vi "Auto Rally Point Calculations.vi"(8 "Rally Point Offset":dbl=24.0, 9 "Depth":dbl=115.0, 10 "Goal Target":T1, 11 "Starting Position":T2) -> (2 "Distance":dbl=294.3908965983833, 3 "Angle":dbl=67.00585386224785)   [LabVIEW 2015]
uses:
  Defense Position.ctl
  Goal Selection.ctl
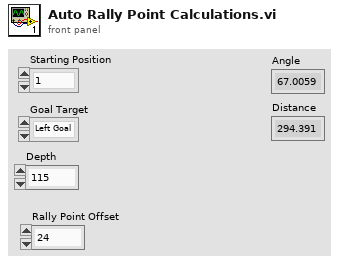
[diagram p1: front panel]
types:
  T1 = typedef "Goal Selection.ctl" = enum16{"Left Goal", "Right Goal"}
  T2 = typedef "Defense Position.ctl" = enum16{"1", "2", "3", "4", "5"}
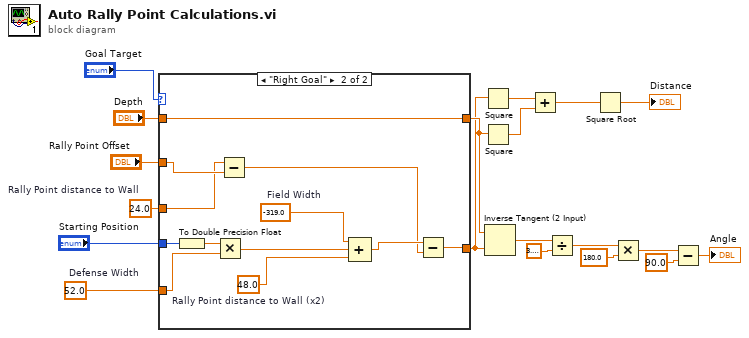
[diagram p0: block diagram]
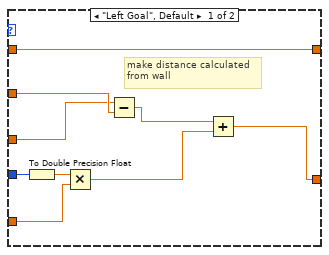
[diagram p2: hidden frame]
diagram:
  w1 = 24.0  # Rally Point distance to Wall
  w12 = 52.0  # Defense Width
  n1 = case shown="\"Right Goal\"" "Goal Target" {
    tunnel: "Depth" -> [w27 w39]
    tunnel: [w23 w31] -> w13
    tunnel: [w27 w39] -> w14
    tunnel: w12 -> [w26 w38]
    tunnel: "Starting Position" -> [w25 w36]
    tunnel: "Rally Point Offset" -> [w21 w33]
    tunnel: w1 -> [w20 w32]
    frame "Left Goal", Default {
      # "make distance calculated\nfrom wall"
      n2 = To Double Precision Float(number=w25) -> (double precision float=w28:dbl)
      n3 = Multiply(x=w28, y=w26) -> (x*y=w24:dbl)
      n4 = Subtract(x=w20, y=w21) -> (x-y=w22:dbl)
      n5 = Add(x=w22, y=w24) -> (x+y=w23:dbl)
    }
    frame "Right Goal" {
      w35 = 48.0  # Rally Point distance to Wall (x2)
      w37 = -319.0  # Field Width
      n6 = To Double Precision Float(number=w36) -> (double precision float=w40:dbl)
      n7 = Multiply(x=w40, y=w38) -> (x*y=w34:dbl)
      n8 = Subtract(x=w32, y=w33) -> (x-y=w29:dbl)
      n9 = Compound Arithmetic op=ADD(w37, w34, w35) -> (w30:dbl)
      n10 = Subtract(x=w30, y=w29) -> (x-y=w31:dbl)
    }
  }
  n11 = Square(x=w13) -> (x^2=w15:dbl)
  n12 = Square(x=w14) -> (x^2=w17:dbl)
  n13 = Inverse Tangent (2 Input)(1:w13, 2:w14) -> (0:w9:dbl)
  n14 = Add(x=w15, y=w17) -> (x+y=w16:dbl)
  n15 = Divide(x=w9, y=3.141592653589793) -> (x/y=w7:dbl)
  n16 = Square Root(x=w16) -> (sqrt(x)=→"Distance":dbl)
  n17 = Multiply(x=w7, y=180.0) -> (x*y=w5:dbl)
  n18 = Subtract(x=w5, y=90.0) -> (x-y=→"Angle":dbl)
